vi "Vision Research Phantom Series PhFile PhGetWriteCineFileProgress.vi"(0 "CH [in]":u32, 5 "Error In (no error)":errorcluster) -> (14 "CH [out]":u32, 15 "pProgressPercent [out]":u32, 19 "Error Out":errorcluster)   [LabVIEW 2013, in "VRI.lvlib"]
doc: "PhGetWriteCineFileProgress\nHRESULT PhGetWriteCineFileProgress(CINEHANDLE CH, PUINT pProgressPercent);\n\nParameters\nCH [in]\n Cine handle.\npProgressPercent [out]\n Pointer where to store current progress percent.\n\nReturn Value\nThe function returns ERR_Ok in case of success or an error code, otherwise. To get extended error information call PhGetErrorMessage.\n\nRemarks\nReturns current save progress for the input cine.\nIt can be called for either an asynchronous or a synchronous write cine operation. However, please note that for a synchronous save operation the thread the save operation has been launched on is expected to be different from the thread this function is called from.\n\nRequired Header\nPhFile.h"
uses:
  VRI.lvlib
  Phantom DLLs/PhFile.Dll
panel:
  # "For instructions on the use of this VI, press Ctrl+H to display the help window and move the mouse over the icon, controls, and indicators"
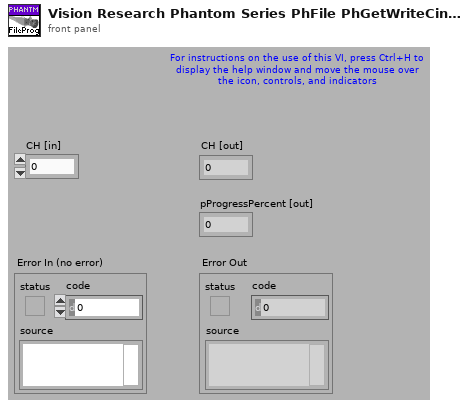
[diagram p1: front panel]
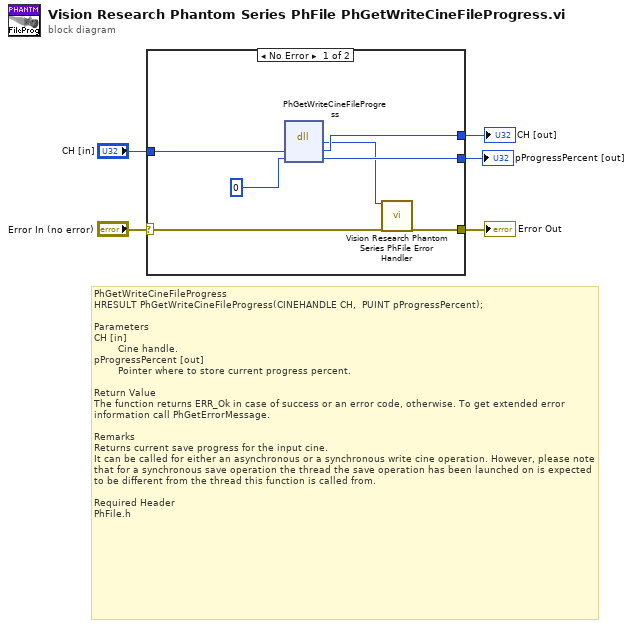
[diagram p0: block diagram]
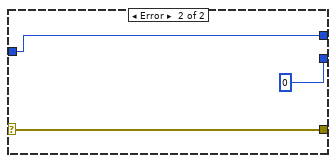
[diagram p2: hidden frame]
diagram:
  # "PhGetWriteCineFileProgress\nHRESULT PhGetWriteCineFileProgress(CINEHANDLE CH,  PUINT pProgressPercent);\n\nParameters\nCH [in]\n\t       Cine handle.\npProgressPercent [out]\n\t       Pointer where to store current progress percent.\n\nReturn Value\nThe function returns ERR_Ok in case of success or an error code, otherwise. To get extended error information call PhGetErrorMessage.\n\nRemarks\nReturns current save progress for the input cine.\nIt can be called for either an asynchronous or a synchronous write cine operation. However, please note that for a synchronous save operation the thread the save operation has been launched on is expected to be different from the thread this function is called from.\n\nRequired Header\nPhFile.h"
  n1 = case shown="No Error" "Error In (no error)" {
    selector: "Error In (no error)" -> [w12 w15]
    tunnel: [w11 w15] -> w4
    tunnel: "CH [in]" -> [w10 w13]
    tunnel: [w9 0] -> w2
    tunnel: [w8 w13] -> w1
    frame No Error {
      n2 = dll-call lib="C:/Projects/SDK/64-bit/Vision Research Phantom Series Labview Driver/Phantom DLLs/PhFile.dll" fn="PhGetWriteCineFileProgress"("CH"=w10, "pProgressPercent"=0) -> ("HRESULT"=w6:i32, "CH"=w8:u32, "pProgressPercent"=w9:u32)  [unwired: 3 in, 2 out]
      n3 = call "Vision Research Phantom Series PhFile Error Handler.vi"("Error Code (0)"=w6, "Error In (no error)"=w12) -> ("Error Out"=w11:errorcluster)  [unwired: 17 out]
    }
    frame Error {
    }
  }
  "Error Out" <- w4
  "pProgressPercent [out]" <- w2
  "CH [out]" <- w1
